vi "Actor Last Ack Decorator.vi"(9 "Nested Error":errorcluster, 10 "Nested Actor":refnum<class "Actor.lvclass">, 11 "Dev Actor in":refnum<class "Dev Actor.lvclass">) -> (0 "error out":errorcluster, 3 "Dev Actor out":refnum<class "Dev Actor.lvclass">)   [LabVIEW 2021, in "Dev Actor.lvlib" / "Dev Actor.lvclass"]
uses:
  Dev Actor.lvclass
  src/LVCAM/LVCAM/Actor/Actor.lvclass
  Dev Actor.lvclass/Dev Actor.ctl
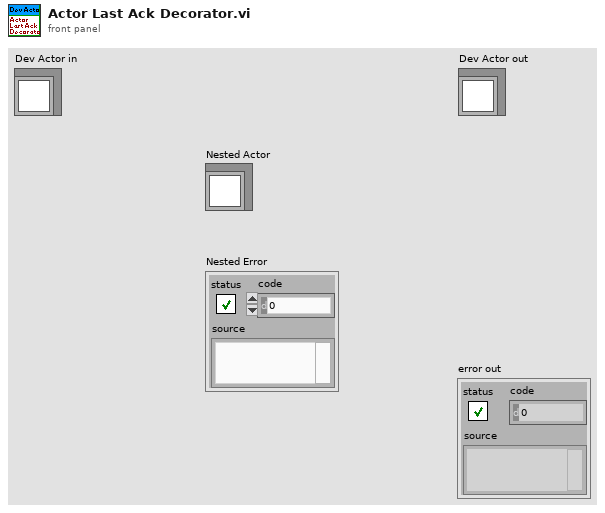
[diagram p1: front panel]
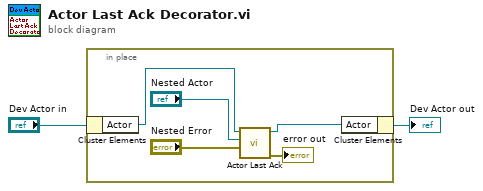
[diagram p0: block diagram]
diagram:
  n1 = in-place {
    n2 = in-place-cluster #1("Dev Actor in") -> ("Actor"=w7:refnum<class "Actor.lvclass">)
    n3 = call-dynamic "Actor Last Ack.vi"("Nested Error"="Nested Error", "Nested Actor"="Nested Actor", "Actor Last Ack in"=w7) -> ("error out"=→"error out":errorcluster, "Actor Last Ack out"=w6:refnum<class "Actor.lvclass">)  [unwired: 7 in]
    n4 = in-place-cluster #1("Actor"=w6) -> (→"Dev Actor out":refnum<class "Dev Actor.lvclass">)
  }
